vi "AO_Amplitude_Pourcent.vi"(8 "error in":errorcluster, 10 "Action":enum16{"Init", "Write", "Read"}(ring), 11 "AO | %":dbl[](array[slide]) min=0.0 max=100.0 step=1.0 scale=0.0..100.0) -> (0 "error out":errorcluster, 3 "AO | %":dbl[](array[slide]) min=0.0 max=100.0 step=1.0 scale=0.0..100.0)   [LabVIEW 2025]
doc: "Functional Global Variable:\n- Write the value into the memory \nor\n- Read the value from the memory"
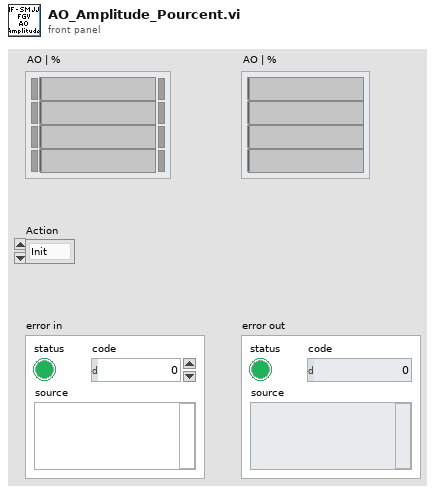
[diagram p1: front panel]
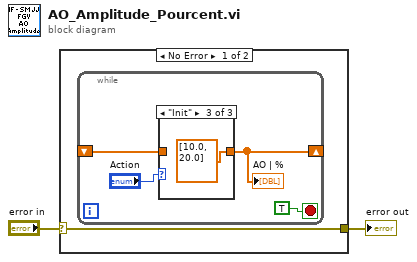
[diagram p0: block diagram]
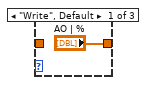
[diagram p2: hidden frame]
diagram:
  n1 = case shown="No Error" "error in" {
    selector: "error in" -> [w3 w11]
    tunnel: [w3 w11] -> w1
    frame No Error {
      n2 = while {
        shift-right: [w4] -> _
        shift-left: _ -> [w5]
        stop <- TRUE stop-if-true
        n3 = case shown="\"Init\"" "Action" {
          tunnel: w5 -> [_ w9 _]
          tunnel: ["AO | %" w9 dbl[] [10.0, 20.0] ("AO | %")] -> w4
          frame "Write", Default {
          }
          frame "Read" {
          }
          frame "Init" {
          }
        }
        "AO | %" <- w4
      }
    }
    frame Error {
    }
  }
  "error out" <- w1
